vi "Read Full Configuration.vi"(8 "error in":errorcluster, 11 "Configuration in":refnum<class "Configuration.lvclass">) -> (0 "error out":errorcluster, 2 "All Tags":string[](array[string]), 3 "Configuration out":refnum<class "Configuration.lvclass">)   [LabVIEW 2019, in "Configuration.lvlib" / "Configuration.lvclass"]
uses:
  Configuration.lvclass
  Configuration.lvclass/Configuration.ctl
  <vilib>/Utility/config.llb/Read Key (String).vi
  <vilib>/Utility/config.llb/NI_LVConfig.lvlib
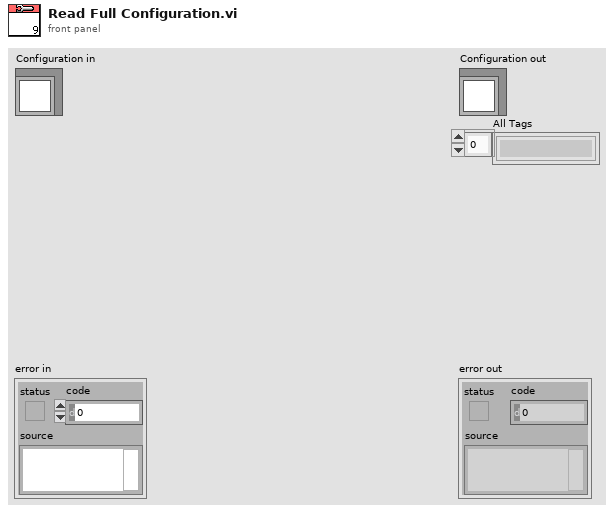
[diagram p1: front panel]
types:
  T1 = typedef "NI_LVConfig.lvlib/Config Data RefNum.ctl" = refnum<k1>
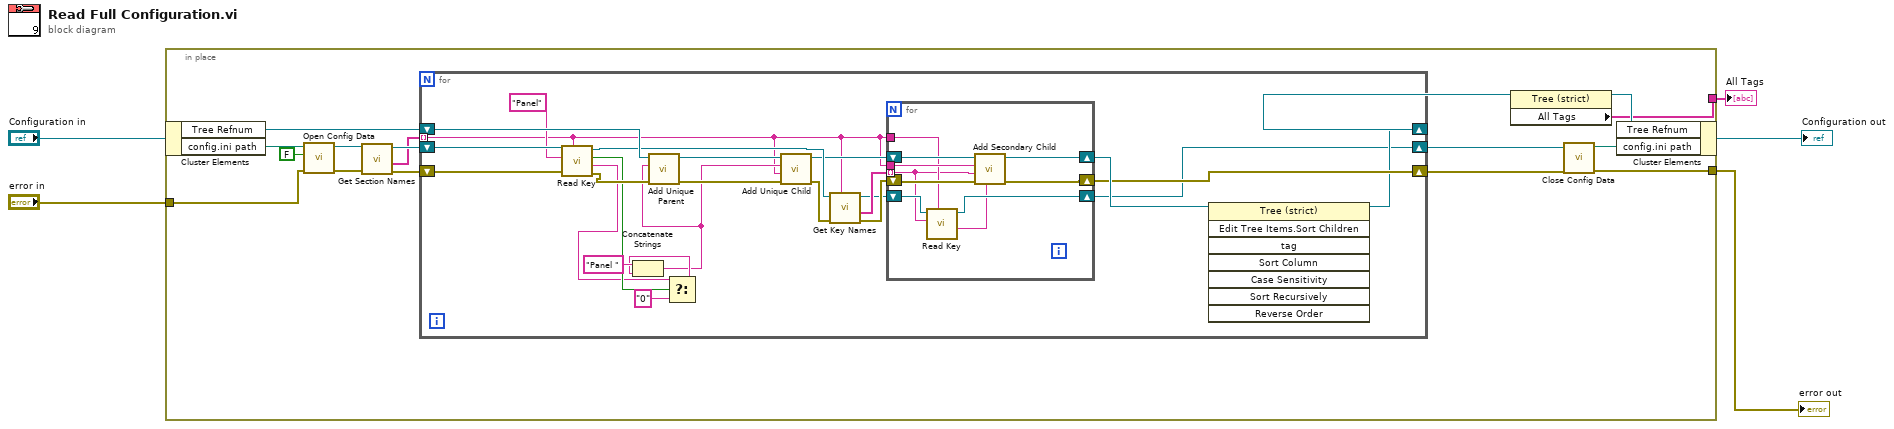
[diagram p0: block diagram]
diagram:
  n1 = in-place {
    in-place-border: "error in" -> [w16]
    in-place-border: [w15] -> w2
    in-place-border: [w6] -> w1
    n2 = in-place-cluster #1("Configuration in") -> ("Tree Refnum"=w10:refnum<vi>, "config.ini path"=w21:path)
    n3 = call <vilib>:"Open Config Data.vi"("error in (no error)"=w16, "create file if necessary (T)"=FALSE, "configuration file path"=w21) -> ("error out"=w18:errorcluster, "refnum"=w17:T1)  [unwired: 6 in, 1 out]
    n4 = call <vilib>:"Get Section Names.vi"("error in (no error)"=w18, "refnum"=w17) -> ("error out"=w13:errorcluster, "section names"=w9:string[], "refnum out"=w14:T1)  [unwired: 7 in]
    n5 = for {
      shift-right: [w23] -> w12
      shift-left: w14 -> [w45]
      shift-right: [w30] -> w11
      shift-left: w13 -> [w44]
      shift-right: [w25] -> w8
      shift-left: w10 -> [w43]
      tunnel: w9 -> [w22] mode=indexing
      n6 = call-poly <vilib>:"Read Key.vi"("section"=w22, "error in (no error)"=w44, "key"="Panel", "refnum"=w45) -> ("error out"=w40:errorcluster, "value"=w26:string, "found?"=w38:bool, "refnum out"=w36:T1)  [unwired: 4 in]
      n7 = Select(t=w26, s=w38, f="0") -> (s? t:f=w28:string)
      n8 = Concatenate Strings("Panel " ("string"), w28) -> (w27:string)
      n9 = call "Add Unique Parent.vi"("error in"=w40, "String"=w27, "Tree Refnum in"=w43) -> ("error out"=w41:errorcluster, "Tree Refnum out"=w42:refnum<vi>)  [unwired: 7 in]
      n10 = call "Add Unique Child.vi"("error in"=w41, "Child"=w22, "Parent"=w27, "Tree Refnum in"=w42) -> ("error out"=w35:errorcluster, "Tree Refnum out"=w34:refnum<vi>)  [unwired: 6 in]
      n11 = call <vilib>:"Get Key Names.vi"("section"=w22, "error in (no error)"=w35, "refnum"=w36) -> ("error out"=w31:errorcluster, "key names"=w32:string[], "refnum out"=w24:T1)  [unwired: 5 in, 1 out]
      n12 = for {
        shift-right: [w54] -> w33
        shift-left: w34 -> [w55]
        shift-right: [w53] -> w30
        shift-left: w31 -> [w52]
        tunnel: w32 -> [w47] mode=indexing
        tunnel: w22 -> [w51]
        shift-right: [w49] -> w23
        shift-left: w24 -> [w50]
        tunnel: w22 -> [w48]
        n13 = call-poly <vilib>:"Read Key.vi"("section"=w48, "key"=w47, "refnum"=w50) -> ("value"=w46:string, "refnum out"=w49:T1)  [unwired: 5 in, 2 out]
        n14 = call "Add Secondary Child.vi"("Value"=w46, "error in"=w52, "Child"=w47, "Parent"=w51, "Tree Refnum in"=w55) -> ("error out"=w53:errorcluster, "Tree Refnum out"=w54:refnum<vi>)  [unwired: 5 in]
      }
      n15 = invoke class="Tree (strict)" method="Edit Tree Items.Sort Children"(reference=w33) -> (reference out=w25:refnum<vi>)  [unwired: 7 in, 7 out]
    }
    n16 = property class="Tree (strict)"(reference=w8) -> (reference out=w7:refnum<vi>, "All Tags"=w6:string[])  [unwired: 1 in, 1 out]
    n17 = call <vilib>:"Close Config Data.vi"("error in (no error)"=w11, "refnum"=w12) -> ("error out"=w15:errorcluster, "file path"=w20:path)  [unwired: 8 in]
    n18 = in-place-cluster #1("Tree Refnum"=w7, "config.ini path"=w20) -> (→"Configuration out":refnum<class "Configuration.lvclass">)
  }
  "error out" <- w2
  "All Tags" <- w1
